vi "Test Launching.vi"() -> ()   [LabVIEW 2011]
uses:
  HW IO/Test Set Definition.ctl
panel:
  out "GetTestSetDef":T1={"General"={"ID"=0, "Model"="", "Dual Port?"=FALSE, "Options"="", "Options"={"E"=FALSE, "K"=FALSE, "H"=FALSE, "W"=FALSE, "F"=FALSE}, "Cal File"=path ""}, "Receiver"={"Fstart, MHz"=0.0, "Fstop MHz"=0.0, "Fstep MHz"=0.0, "IF, MHz"=0.0}, "RX Band"={"Fstart, MHz"=0.0, "Fstop MHz"=0.0}, "TX 1"={"Fstart, MHz"=0.0, "Fstop MHz"=0.0, "Pmax, dBm"=0.0, "Pstep, dB"=0.0}, "TX 2"={"Fstart, MHz"=0.0, "Fstop MHz"=0.0, "Pmax, dBm"=0.0, "Pstep, dB"=0.0}, "Low-side?"=TRUE}
  out "GetCalInfo":T2
  out "GetError - HW Error":errorcluster
  out "Launch HW TestSetDef":T1={"General"={"ID"=0, "Model"="", "Dual Port?"=FALSE, "Options"="", "Options"={"E"=FALSE, "K"=FALSE, "H"=FALSE, "W"=FALSE, "F"=FALSE}, "Cal File"=path ""}, "Receiver"={"Fstart, MHz"=0.0, "Fstop MHz"=0.0, "Fstep MHz"=0.0, "IF, MHz"=0.0}, "RX Band"={"Fstart, MHz"=0.0, "Fstop MHz"=0.0}, "TX 1"={"Fstart, MHz"=0.0, "Fstop MHz"=0.0, "Pmax, dBm"=0.0, "Pstep, dB"=0.0}, "TX 2"={"Fstart, MHz"=0.0, "Fstop MHz"=0.0, "Pmax, dBm"=0.0, "Pstep, dB"=0.0}, "Low-side?"=TRUE}
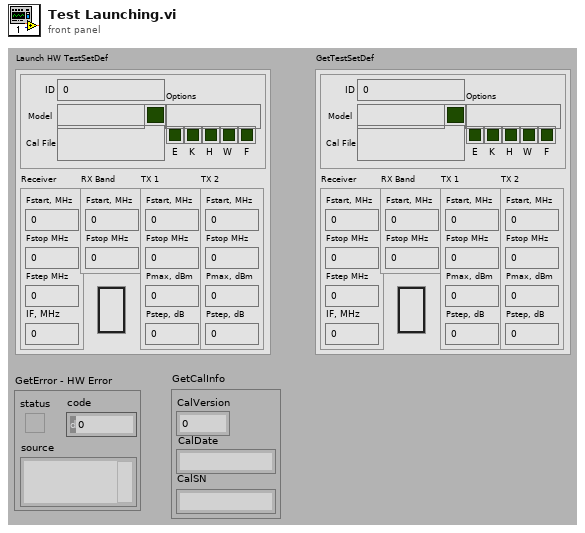
[diagram p1: front panel]
types:
  T1 = typedef "Test Set Definition.ctl" = cluster{"General":cluster{"ID":u32, "Model":string, "Dual Port?":bool, "Options":string, "Options":cluster{"E":bool, "K":bool, "H":bool, "W":bool, "F":bool}, "Cal File":path}, "Receiver":cluster{"Fstart, MHz":dbl, "Fstop MHz":dbl, "Fstep MHz":dbl, "IF, MHz":dbl}, "RX Band":cluster{"Fstart, MHz":dbl, "Fstop MHz":dbl}, "TX 1":cluster{"Fstart, MHz":dbl, "Fstop MHz":dbl, "Pmax, dBm":dbl, "Pstep, dB":dbl}, "TX 2":cluster{"Fstart, MHz":dbl, "Fstop MHz":dbl, "Pmax, dBm":dbl, "Pstep, dB":dbl}, "Low-side?":bool}
  T2 = cluster{"CalVersion":u8, "CalDate":string, "CalSN":string}
  T3 = cluster{"version":u8, "date":string, "serial number":string, "datestamp":dbl, "validCal?":bool}
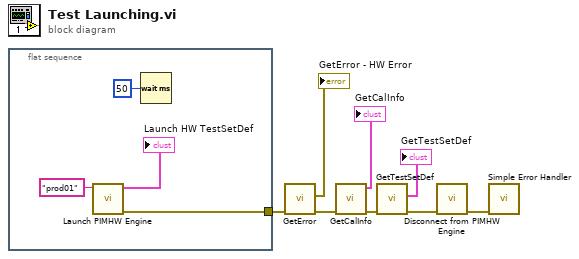
[diagram p0: block diagram]
diagram:
  n1 = flat-sequence {
    tunnel: [w12] -> w8
    frame #0 {
      n2 = call "Launch PIMHW Engine.vi"("host (localhost)"="prod01" ("pimhw\nhost\n(emtpy\nfor localhost)")) -> ("error out"=w12:errorcluster, "TestSetDef"=→"Launch HW TestSetDef":T1)  [unwired: 6 in, 3 out]
      n3 = Wait (ms)(milliseconds to wait=u32 50) -> ()  [unwired: 1 out]
    }
  }
  n4 = call "GetError.vi"("error in (no error)"=w8) -> ("error out"=w7:errorcluster, "HW Error"=→"GetError - HW Error":errorcluster)  [unwired: 1 in, 8 out]
  n5 = call "GetCalInfo.vi"("error in (no error)"=w7) -> ("error out"=w6:errorcluster, "CalInfo"=→"GetCalInfo":T3)  [unwired: 2 in, 7 out]
  n6 = call "GetTestSetDef.vi"("error in (no error)"=w6) -> ("error out"=w2:errorcluster, "TestSetDef"=→"GetTestSetDef":T1)  [unwired: 2 in, 7 out]
  n7 = call "Disconnect from PIMHW Engine.vi"("error in (no error)"=w2) -> ("error out"=w1:errorcluster)  [unwired: 10 in]
  n8 = call <vilib>:"Simple Error Handler.vi"("error in (no error)"=w1) -> ()  [unwired: 1 in, 8 out]
